vi "Check Solution Exists.vi"(8 "Error In":errorcluster, 10 "Solution Label":string, 11 "Author Initials":string) -> (0 "Error Out":errorcluster, 3 "Solution Label Duplicate?":bool)   [LabVIEW 2020]
uses:
  Data Handling Operations/Data Clusters/Database Information.ctl
  Data Handling Operations/Data Clusters/Layer Information Cluster.ctl
  <vilib>/addons/database/Connection.llb/Conn ObjectReference.ctl
  <vilib>/addons/database/NI_Database_API.lvlib
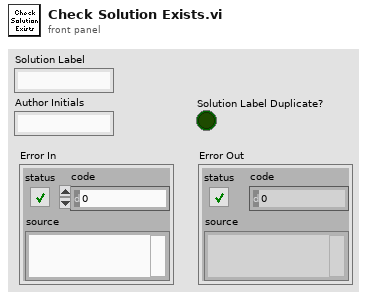
[diagram p1: front panel]
types:
  T1 = typedef "Database Information.ctl" = cluster{"Database Extracted Information":cluster{"Author Information":cluster{"Author Initials":string, "Author ID":i32}, "Batch Information":cluster{"Batch Label":string, "Batch ID":i32}, "Current Layer Solution":cluster{"Solution Label":string, "Solution ID":i32}, "Current Layer ID":i32, "Current Layer Solvent Inf":cluster{"Solvent Name":string, "Solvent ID":i32, "Ratio":dbl}[], "Current Layer Material Inf":cluster{"Material Name":string, "Material ID":i32, "Ratio":dbl}[], "Added New Solution to DB?":bool, "Added New Batch to DB?":bool}, "Database Write Information":cluster{"Author Initials":string, "Batch Label":string, "Layer Information Array":T2[], "JV Measurement Array":cluster{"Pixel Label":string, "Voc (V) ":dbl, "Jsc (A/m^2) ":dbl, "Efficiency (%)":dbl, "FF (%)":dbl, "Rs (O m^2)":dbl, "Rsh (O m^2)":dbl, "Light Power Density (W/m^2)":dbl, "Pixel Area (m^2)":dbl, "JV Measurement Date":string, "JV Measurement File":string, "Measurement Comments":string}[]}, "Database Connection":T3}
  T2 = typedef "Layer Information Cluster.ctl" = cluster{"Solution Information Cluster":cluster{"Solution Label":string, "Solution Concentration (mg/ml)":dbl, "Solution Comments ":string, "Solution Volume (ul) ":dbl, "Solution Date ":string, "Solution Descriptor ":string, "Solution Stir Temperature ºC ":dbl, "Solution Stir Time (kr) ":dbl, "Solution In Glovebox":bool, "Solvent Array":cluster{"Solvent Name":string, "Ratio":dbl}[], "Material Array":cluster{"Material Name":string, "Ratio":dbl}[]}, "Layer Type":u16, "Deposition Method":u16, "Layer Annealing":bool, "General Deposition Parameters":cluster{"Thickness (nm)":dbl, "Comments":string, "Material Name":string}, "Blade Coating Parameters":cluster{"Thickness (nm)":dbl, "Initial Blade Speed (mm/s)":dbl, "Speed Gradient":bool, "Final Blade Speed (mm/s)":dbl, "Blade Gap (um)":dbl, "Droplet Volume (ul)":dbl, "Subsequent Layers":dbl, "Inside Glovebox":bool, "Comments":string, "Blade Temperature ºC":dbl}, "Spin Coating Parameters":cluster{"Thickness (nm)":dbl, "Spin Speed (rpm)":dbl, "Dynamic Deposition":bool, "Spin Acceleration":dbl, "Spin Time (s)":dbl, "Droplet Volume (ul)":dbl, "Subsequent Layers":dbl, "Inside Glovebox":bool, "Comments":string}, "Thermal Evaporation Parameters":cluster{"Deposition Rate (A/s)":dbl, "Thickness (nm)":dbl, "Comments":string, "Material Name":string, "Sample Rotation":bool}, "Layer Date 'YYYY-MM-DD'":string, "Annealing Time (kr)":dbl, "Annealing Temperature (ºC)":dbl, "Deposition Method Flags":cluster{"Blade Coating":bool, "General ":bool, "Solution":bool, "Spin Coating":bool, "Thermal Evaporation":bool}}
  T3 = typedef "NI_Database_API.lvlib/Conn ObjectReference.ctl" = refnum<k1>
  T4 = cluster{"Author Initials":string, "Author ID":i32}
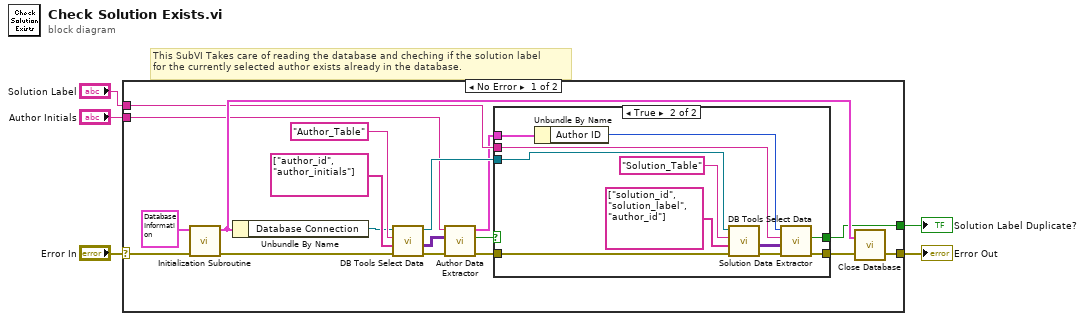
[diagram p0: block diagram]
diagram:
  # "This SubVI Takes care of reading the database and cheching if the solution label\nfor the currently selected author exists already in the database."
  n1 = case shown="No Error" "Error In" {
    selector: "Error In" -> [w23 w36]
    tunnel: [w22 w36] -> w4
    tunnel: "Solution Label" -> [w19 _]
    tunnel: "Author Initials" -> [w9 _]
    tunnel: [w6 _] -> w1
    frame No Error {
      n2 = call "Initialization Subroutine.vi"("Error In"=w23, "Database Full Information In"=T1 {"Database Extracted Information"={"Author Information"={"Author Initials"="", "Author ID"=0}, "Batch Information"={"Batch Label"="", "Batch ID"=0}, "Current Layer Solution"={"Solution Label"="", "Solution ID"=0}, "Current Layer ID"=0, "Current Layer Solvent Inf"=[], "Current Layer Material Inf"=[], "Added New Solution to DB?"=FALSE, "Added New Batch to DB?"=FALSE}, "Database Write Information"={"Author Initials"="", "Batch Label"="", "Layer Information Array"=[], "JV Measurement Array"=[]}, "Database Connection"=refnum} ("input cluster")) -> ("Error Out"=w14:errorcluster, "Database Full Information Out"=w21:T1)  [unwired: 8 in]
      n3 = Unbundle By Name(w21) -> ("Database Connection"=w12:T3)
      n4 = call <vilib>:"DB Tools Select Data.vi"("error in (no error)"=w14, "columns"=string[] ["author_id", "author_initials"], "table"="Author_Table", "connection reference"=w12) -> ("error out"=w16:errorcluster, "data"=w17:variant[][], "connection reference out"=w11:T3)  [unwired: 2 in]
      n5 = call "Author Data Extractor.vi"("Error In"=w16, "Author Data"=w17, "Author Initials"=w9) -> ("Error Out"=w13:errorcluster, "Exists?"=w7:bool, "Author Information"=w8:T4)  [unwired: 6 in]
      n6 = case shown="True" w7 {
        tunnel: [w24 w31] -> w20
        tunnel: w19 -> [_ w30]
        tunnel: w13 -> [w24 w29]
        tunnel: w11 -> [_ w28]
        tunnel: w8 -> [_ w27]
        tunnel: [_ w25] -> w6
        frame False {
        }
        frame True {
          n7 = Unbundle By Name(w27) -> ("Author ID"=w26:i32)
          n8 = call <vilib>:"DB Tools Select Data.vi"("error in (no error)"=w29, "columns"=string[] ["solution_id", "solution_label", "author_id"], "table"="Solution_Table", "connection reference"=w28) -> ("error out"=w33:errorcluster, "data"=w32:variant[][])  [unwired: 2 in, 1 out]
          n9 = call "Solution Data Extractor.vi"("Error In"=w33, "Solution Data"=w32, "Solution Label"=w30, "Author ID"=w26) -> ("Error Out"=w31:errorcluster, "Exists?"=w25:bool)  [unwired: 5 in, 1 out]
        }
      }
      n10 = call "Close Database.vi"("Error In"=w20, "Database Full Information In"=w21) -> ("Error Out"=w22:errorcluster)  [unwired: 1 in]
    }
    frame Error {
    }
  }
  "Error Out" <- w4
  "Solution Label Duplicate?" <- w1
